vi "Drive Controller.vi"(8 "error in":errorcluster) -> ()   [LabVIEW 2016]
doc: "This VI executes continuously carrying out the current operation and responding to updates or new operation requests. It will often contain the timing or control code that is difficult to place directly in TeleOp. This VI generally opens all sensors and motors and isolates the rest of the robot code from knowing implementation details of how the operations are carried out."
uses:
  Drive Setpoints.ctl
  Drive Operations.ctl
  <vilib>/Rock Robotics/WPI/SafetyOutput/WPI_SafetyOutputConfigMenu.ctl
  <vilib>/Rock Robotics/WPI/Solenoid/WPI_SolenoidChannel.ctl
  <vilib>/Rock Robotics/SystemInterfaces/DIO/FPGA_DIOChannel.ctl
  <vilib>/Rock Robotics/WPI/ThirdParty/CanMotor/TalonSRX/WPI_CANTalonSRX_APIControlMode.ctl
  <vilib>/Rock Robotics/SystemInterfaces/AI/FPGA_AIChannel.ctl
  <vilib>/Rock Robotics/SystemInterfaces/spilib/spi_bus.ctl
  <vilib>/Rock Robotics/WPI/Solenoid/WPI_SolenoidValue.ctl
  <vilib>/Rock Robotics/WPI/Solenoid/WPI_SolenoidOpenDouble.vi
  <vilib>/Rock Robotics/WPI/Counter/WPI_CounterDigitalInputToDigitalSource.vi
  <vilib>/Rock Robotics/WPI/RobotDrive/WPI_RobotDriveOpen2MotorWithExistingMotors.vi
  <vilib>/Rock Robotics/WPI/Solenoid/WPI_SolenoidOpenSingle.vi
  <vilib>/Rock Robotics/WPI/ThirdParty/Sensors/Pigeon IMU/CTRE_PigeonIMU_Open_CAN.vi
  <vilib>/Rock Robotics/Network Tables/NT Read Number.vi
  <vilib>/Rock Robotics/WPI/Solenoid/WPI_SolenoidSetEnum.vi
  Drive Published Globals.vi
  <vilib>/Rock Robotics/Network Tables/NT Write Boolean.vi
  <vilib>/Rock Robotics/Network Tables/NT Write Number.vi
  Framework/Robot Global Data.vi
  <vilib>/addons/control/pid/pid.llb/PID (DBL).vi
  <vilib>/Rock Robotics/Network Tables/NT Write String.vi
  <vilib>/addons/control/pid/NI_PID_pid.lvlib
  <vilib>/Rock Robotics/WPI/ThirdParty/Sensors/navX/_Processing Loop/FRIC_navX_Internal_I2C_ProcessingLoop.vi
panel:
  out "Pigeon  Chart 2":dbl(graph)=-34.541015625
  out "Voltage now":dbl=1.910400195
  in  "Fcurving right":dbl=0.0045 format="%#_13g"
  in  "Fcurving left":dbl=0.0045 format="%#_13g"
  out "Vision P tuning threshold":dbl(graph)=6.5
  in  "AverageBits":u8=20
  out "Voltage Graph":dbl(graph)=1.910400195
  out "Voltage":dbl=1.2902830710000002
  in  "Threshold voltage":dbl=1.8
  out "Waveform Chart 2":cluster{"Heading":dbl, "\n\n\npigeon":dbl}(graph)={"Heading"=81.826171875, "\n\n\npigeon"=39.0673828125}
  out "Pigeon angle":dbl
  out "Waveform Chart":cluster{"Distance":dbl, "Distance":dbl}(graph)={"Distance"=9964.75, "Distance"=10153.75}
  in  "PDriveStright":dbl=0.02
  out "Pigeon  Chart":dbl(graph)=-40.1220703125
  in  "P curving factor":dbl=2.0
  in  "Theshold for curve":dbl=9.0
  in  "X resolution":dbl=160.0
  in  "y":dbl=0.15
  in  "PID gains":T1={"proportional gain (Kc)"=0.1, "integral time (Ti, min)"=0.0, "derivative time (Td, min)"=0.0} {"derivative time (Td, min)" format="%.3f"; "integral time (Ti, min)" format="%.3f"; "proportional gain (Kc)" format="%.3f"}
  in  "Score Cutoff":dbl=40.0
  in  "Y stopping threshold":dbl=70.0
  in  "ticks per rotation":dbl=512.0
  in  "Base Speed":dbl=-0.5499999999999999
  in  "P Gear Tuner":dbl=0.5
  in  "Max dist":dbl=1.0
  out "Setpoints":T2(graph)
  out "Current\nCmd":string="Started at  12:31:04.564\nDefault: Reserve,  L 0.0, R 0.0, D 0.000000"
  # "Gear Vision Stuff"
  # "Tip: It may be helpful to observe inputs and sensor values.\nYou may also want to display tuning or debugging controls."
  # "Used to be .25 on comp robot, .3 may work better though"
  # ".02*10 degrees =.2 motor power!!!"
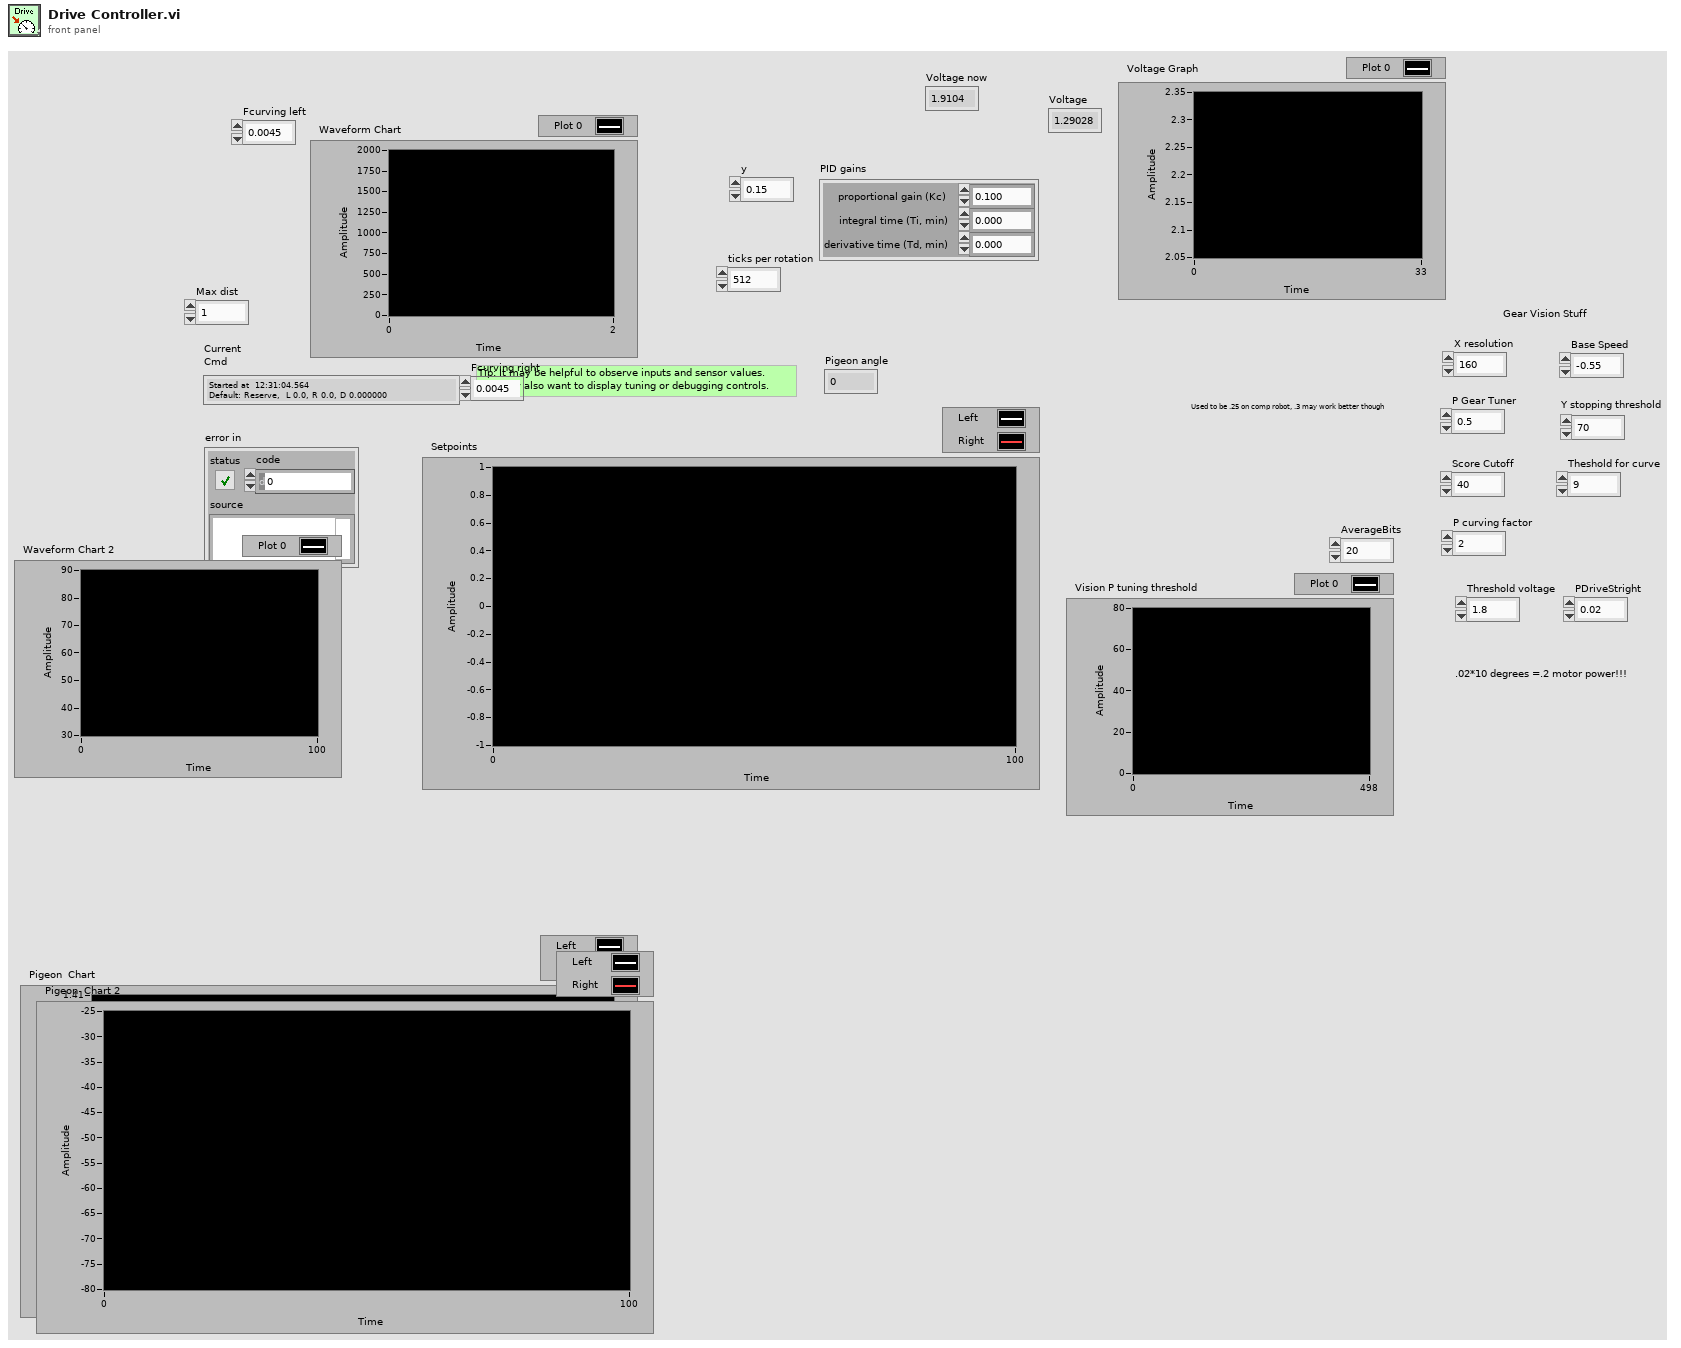
[diagram p1: front panel]
types:
  T1 = cluster{"proportional gain (Kc)":dbl, "integral time (Ti, min)":dbl, "derivative time (Td, min)":dbl}
  T2 = cluster{"Left Setpoint":dbl, "Right Setpoint":dbl}
  T3 = typedef "FPGA_AIChannel.ctl" = enum8{"AI 0", "AI 1", "AI 2", "AI 3", "AI MXP 0", "AI MXP 1", "AI MXP 2", "AI MXP 3", "Invalid"}
  T4 = typedef "WPI_SolenoidChannel.ctl" = enum8{"Solenoid 0", "Solenoid 1", "Solenoid 2", "Solenoid 3", "Solenoid 4", "Solenoid 5", "Solenoid 6", "Solenoid 7", "Invalid"}
  T5 = typedef "WPI_CANTalonSRX_APIControlMode.ctl" = enum8{"Percent VBus", "Speed", "Position", "Slave", "Unchanged / Invalid", "Voltage Compensation", "Current", "Motion Profile", "Motion Magic"}
  T6 = typedef "FPGA_DIOChannel.ctl" = enum8{"DIO 0", "DIO 1", "DIO 2", "DIO 3", "DIO 4", "DIO 5", "DIO 6", "DIO 7", "DIO 8", "DIO 9", "DIO MXP 0", "DIO MXP 1", "DIO MXP 2", "DIO MXP 3", "DIO MXP 4", "DIO MXP 5", "DIO MXP 6", "DIO MXP 7", "DIO MXP 8", "DIO MXP 9", "DIO MXP 10", "DIO MXP 11", "DIO MXP 12", "DIO MXP 13", "DIO MXP 14", "DIO MXP 15", "SPI Port CS1", "SPI Port CS2", "SPI Port CS3", "SPI Port MISO", "SPI Port MOSI", "Invalid"}
  T7 = typedef "spi_bus.ctl" = enum16{"SPI On-Board, CS0", "SPI On-Board, CS1", "SPI On-Board, CS2", "SPI On-Board, CS3", "SPI MXP", "Invalid"}
  T8 = typedef "WPI_SafetyOutputConfigMenu.ctl" = enum16{"Enable", "Disable"}
  T9 = typedef "Drive Setpoints.ctl" = cluster{"Operation":T10, "Left Setpoint":dbl, "Right Setpoint":dbl, "Duration":dbl, "Shift state":i8, "Angle":dbl, "Brake":bool}
  T10 = typedef "Drive Operations.ctl" = enum16{"Reserve", "Read Current", "Immediate", "Drive for Time", "Drive for Distance", "Turn to angle", "Vision Turn", "Vision close distance", "Reset Gyro", "Turn until target", "Brake", "One side PID drive straight", "turn to zero", "DriveStraight"}
  T11 = typedef "WPI_DigitalInputDevRef.ctl" = cluster{"DevStatus":errorcluster, "DIO Channel":T6}
  T12 = typedef "WPI_MotorControlDeviceRef.ctl" = cluster{"DeviceStatus":errorcluster, "Type":T13, "PWM":cluster{"PWM Channel":T14, "DeadBand":T15}, "CAN":cluster{"Device Number":u8, "SetOutput VI Ref":variant, "GetOutput VI Ref":variant, "Enable VI Ref":variant, "Disable VI Ref":variant, "Data":variant}, "Invert":bool}
  T13 = typedef "WPI_MotorControlType.ctl" = enum16{"PWM", "CAN"}
  T14 = typedef "FPGA_DIOPWMChannel.ctl" = enum8{"PWM 0", "PWM 1", "PWM 2", "PWM 3", "PWM 4", "PWM 5", "PWM 6", "PWM 7", "PWM 8", "PWM 9", "PWM MXP 0", "PWM MXP 1", "PWM MXP 2", "PWM MXP 3", "PWM MXP 4", "PWM MXP 5", "PWM MXP 6", "PWM MXP 7", "PWM MXP 8", "PWM MXP 9", "Invalid"}
  T15 = typedef "WPI_PWMDeadband.ctl" = cluster{"Name":string, "maxPositivePwm":i32, "minPositivePwm":i32, "centerPwm":i32, "maxNegativePwm":i32, "minNegativePwm":i32, "angularRange":u16}
  T16 = typedef "WPI_RobotDriveDevRef.ctl" = cluster{"DevStatus":errorcluster, "Motors[]":T12[], "Square Inputs":bool, "Max Output":dbl}
  T17 = typedef "FPGA_CounterEncoderSourceConvertionLVSourceType.ctl" = cluster{"DevStatus":errorcluster, "AnalogTriggerMode?":bool, "DigitalMode":cluster{"DIO Channel":T18}, "AnalogTriggerMode":cluster{"AnalogTriggerIndex":T19, "OutputType":T20}}
  T18 = typedef "FPGA_DIODigitalSourceChannel.ctl" = enum8{"DIO 0", "DIO 1", "DIO 2", "DIO 3", "DIO 4", "DIO 5", "DIO 6", "DIO 7", "DIO 8", "DIO 9", "DIO MXP 0", "DIO MXP 1", "DIO MXP 2", "DIO MXP 3", "DIO MXP 4", "DIO MXP 5", "DIO MXP 6", "DIO MXP 7", "DIO MXP 8", "DIO MXP 9", "DIO MXP 10", "DIO MXP 11", "DIO MXP 12", "DIO MXP 13", "DIO MXP 14", "DIO MXP 15", "Disabled"}
  T19 = typedef "FPGA_AnalogTriggerIndex.ctl" = enum8{"Trig 0", "Trig 1", "Trig 2", "Trig 3", "Trig 4", "Trig 5", "Trig 6", "Trig 7", "Invalid"}
  T20 = typedef "FPGA_AnalogTriggerOutType.ctl" = enum16{"InWindow", "TriggerState", "Rising", "Falling"}
  T21 = typedef "WPI_EncoderDevRef.ctl" = cluster{"DevStatus":errorcluster, "EncoderIndex":T22, "CounterIndex":T23, "DistancePerCount":dbl, "Decoding Type":T24}
  T22 = typedef "FPGA_EncoderIdx.ctl" = enum8{"Enc 0", "Enc 1", "Enc 2", "Enc 3", "Enc 4", "Enc 5", "Enc 6", "Enc 7", "Invalid"}
  T23 = typedef "FPGA_CounterCtrSystemIndex.ctl" = enum8{"Ctr 0", "Ctr 1", "Ctr 2", "Ctr 3", "Ctr 4", "Ctr 5", "Ctr 6", "Ctr 7", "Invalid"}
  T24 = typedef "WPI_EncoderType.ctl" = enum16{"1x", "2x", "4x"}
  T25 = typedef "WPI_SolenoidDevRef.ctl" = cluster{"DevStatus":errorcluster, "Pneumatics Control Module":u8, "Forward Solenoid Channel":T4, "Reverse Solenoid Channel":T4}
  T26 = typedef "Command Status Info.ctl" = cluster{"Name":string, "Status":T27, "notifier out":T28}
  T27 = typedef "Completion Status.ctl" = enum16{"Successful", "Aborted", "Incomplete"}
  T28 = typedef "Completion Notifier.ctl" = refnum<notifier>
  T29 = cluster{"SubSystem Data":T9, cluster{"Start Time (ms)":u32, "Iterations":i32}, cluster{"Command Info":T26, "Description":string, "SubSystem Data":T9, "notifier out":refnum<notifier>, "Subsystem Name":string}}
  T30 = typedef "CTRE_PigeonIMU_DeviceRef.ctl" = cluster{"DeviceStatus":errorcluster, "Device Number":u8, "Type":T31, "Device ID":u32}
  T31 = typedef "CTRE_PigeonIMU_ConnectionType.ctl" = u32
  T32 = typedef "WPI_AnalogChannelDevRef.ctl" = cluster{"DevStatus":errorcluster, "Analog Channel":T3}
  T33 = typedef "WPI_SolenoidValue.ctl" = enum16{"Off", "On", "Forward", "Reverse"}
  T34 = typedef "CTRE_PigeonIMU_GlobalStatus.ctl" = cluster{"PigeonState":T35, "FusedHeading":cluster{"Heading":dbl, "Valid?":bool, "Fusing?":bool}, "YPR":cluster{"Yaw":dbl, "Pitch":dbl, "Roll":dbl}, "Compass":cluster{"Heading":dbl, "Magnitude":dbl, "Absolute Heading":dbl}, "Accelerometer":cluster{"Biased":cluster{"X":i16, "Y":i16, "Z":i16, "Norm":i16}, "Angles":cluster{"XZ Tilt":dbl, "YZ Tilt":dbl, "XY Tilt":dbl}}, "Magnetometer":cluster{"Raw":cluster{"X":i16, "Y":i16, "Z":i16}, "Biased":cluster{"X":i16, "Y":i16, "Z":i16}}, "Gyro":cluster{"X":dbl, "Y":dbl, "Z":dbl, "Norm":dbl}, "6D Quaternian":cluster{"W":dbl, "X":dbl, "Y":dbl, "Z":dbl}, "Temp. (C)":dbl, "UpTime":u32, "StartupStatus":cluster{"ResetCount":i32, "ResetFlags":i32, "FirmwareVersion":i32, "HasReset?":bool}, "Calibration":cluster{"CurrentMode":T36, "LastCalError":i32, "CalBooting?":bool}, "CAN Error":errorcluster, "AccumGyro":cluster{"X":dbl, "Y":dbl, "Z":dbl}, "Usage Frame":u32}
  T35 = typedef "CTRE_PigeonIMU_PigeonState.ctl" = enum16{"NoComm", "Initializing", "Ready", "UserCalibration"}
  T36 = typedef "CTRE_PigeonIMU_CalibrationMode.ctl" = u16
  T37 = cluster{"Left":dbl, "Top":dbl, "Right":dbl, "Bottom":dbl}
  T38 = cluster{"SubSystem Data":T9, cluster{"Start Time (ms)":u32, "Iterations":i32}, "Default Command Arguments":cluster{"Command Info":T26, "Description":string, "SubSystem Data":T9, "notifier out":refnum<notifier>, "Subsystem Name":string}}
  T39 = typedef "WPI_DriverStationRobotMode2.ctl" = enum16{"Autonomous Disabled", "Autonomous Enabled", "Teleop Disabled", "Teleop Enabled", "Disconnected", "Finish", "Test Disabled", "Test Enabled", "Emergency Stopped"}
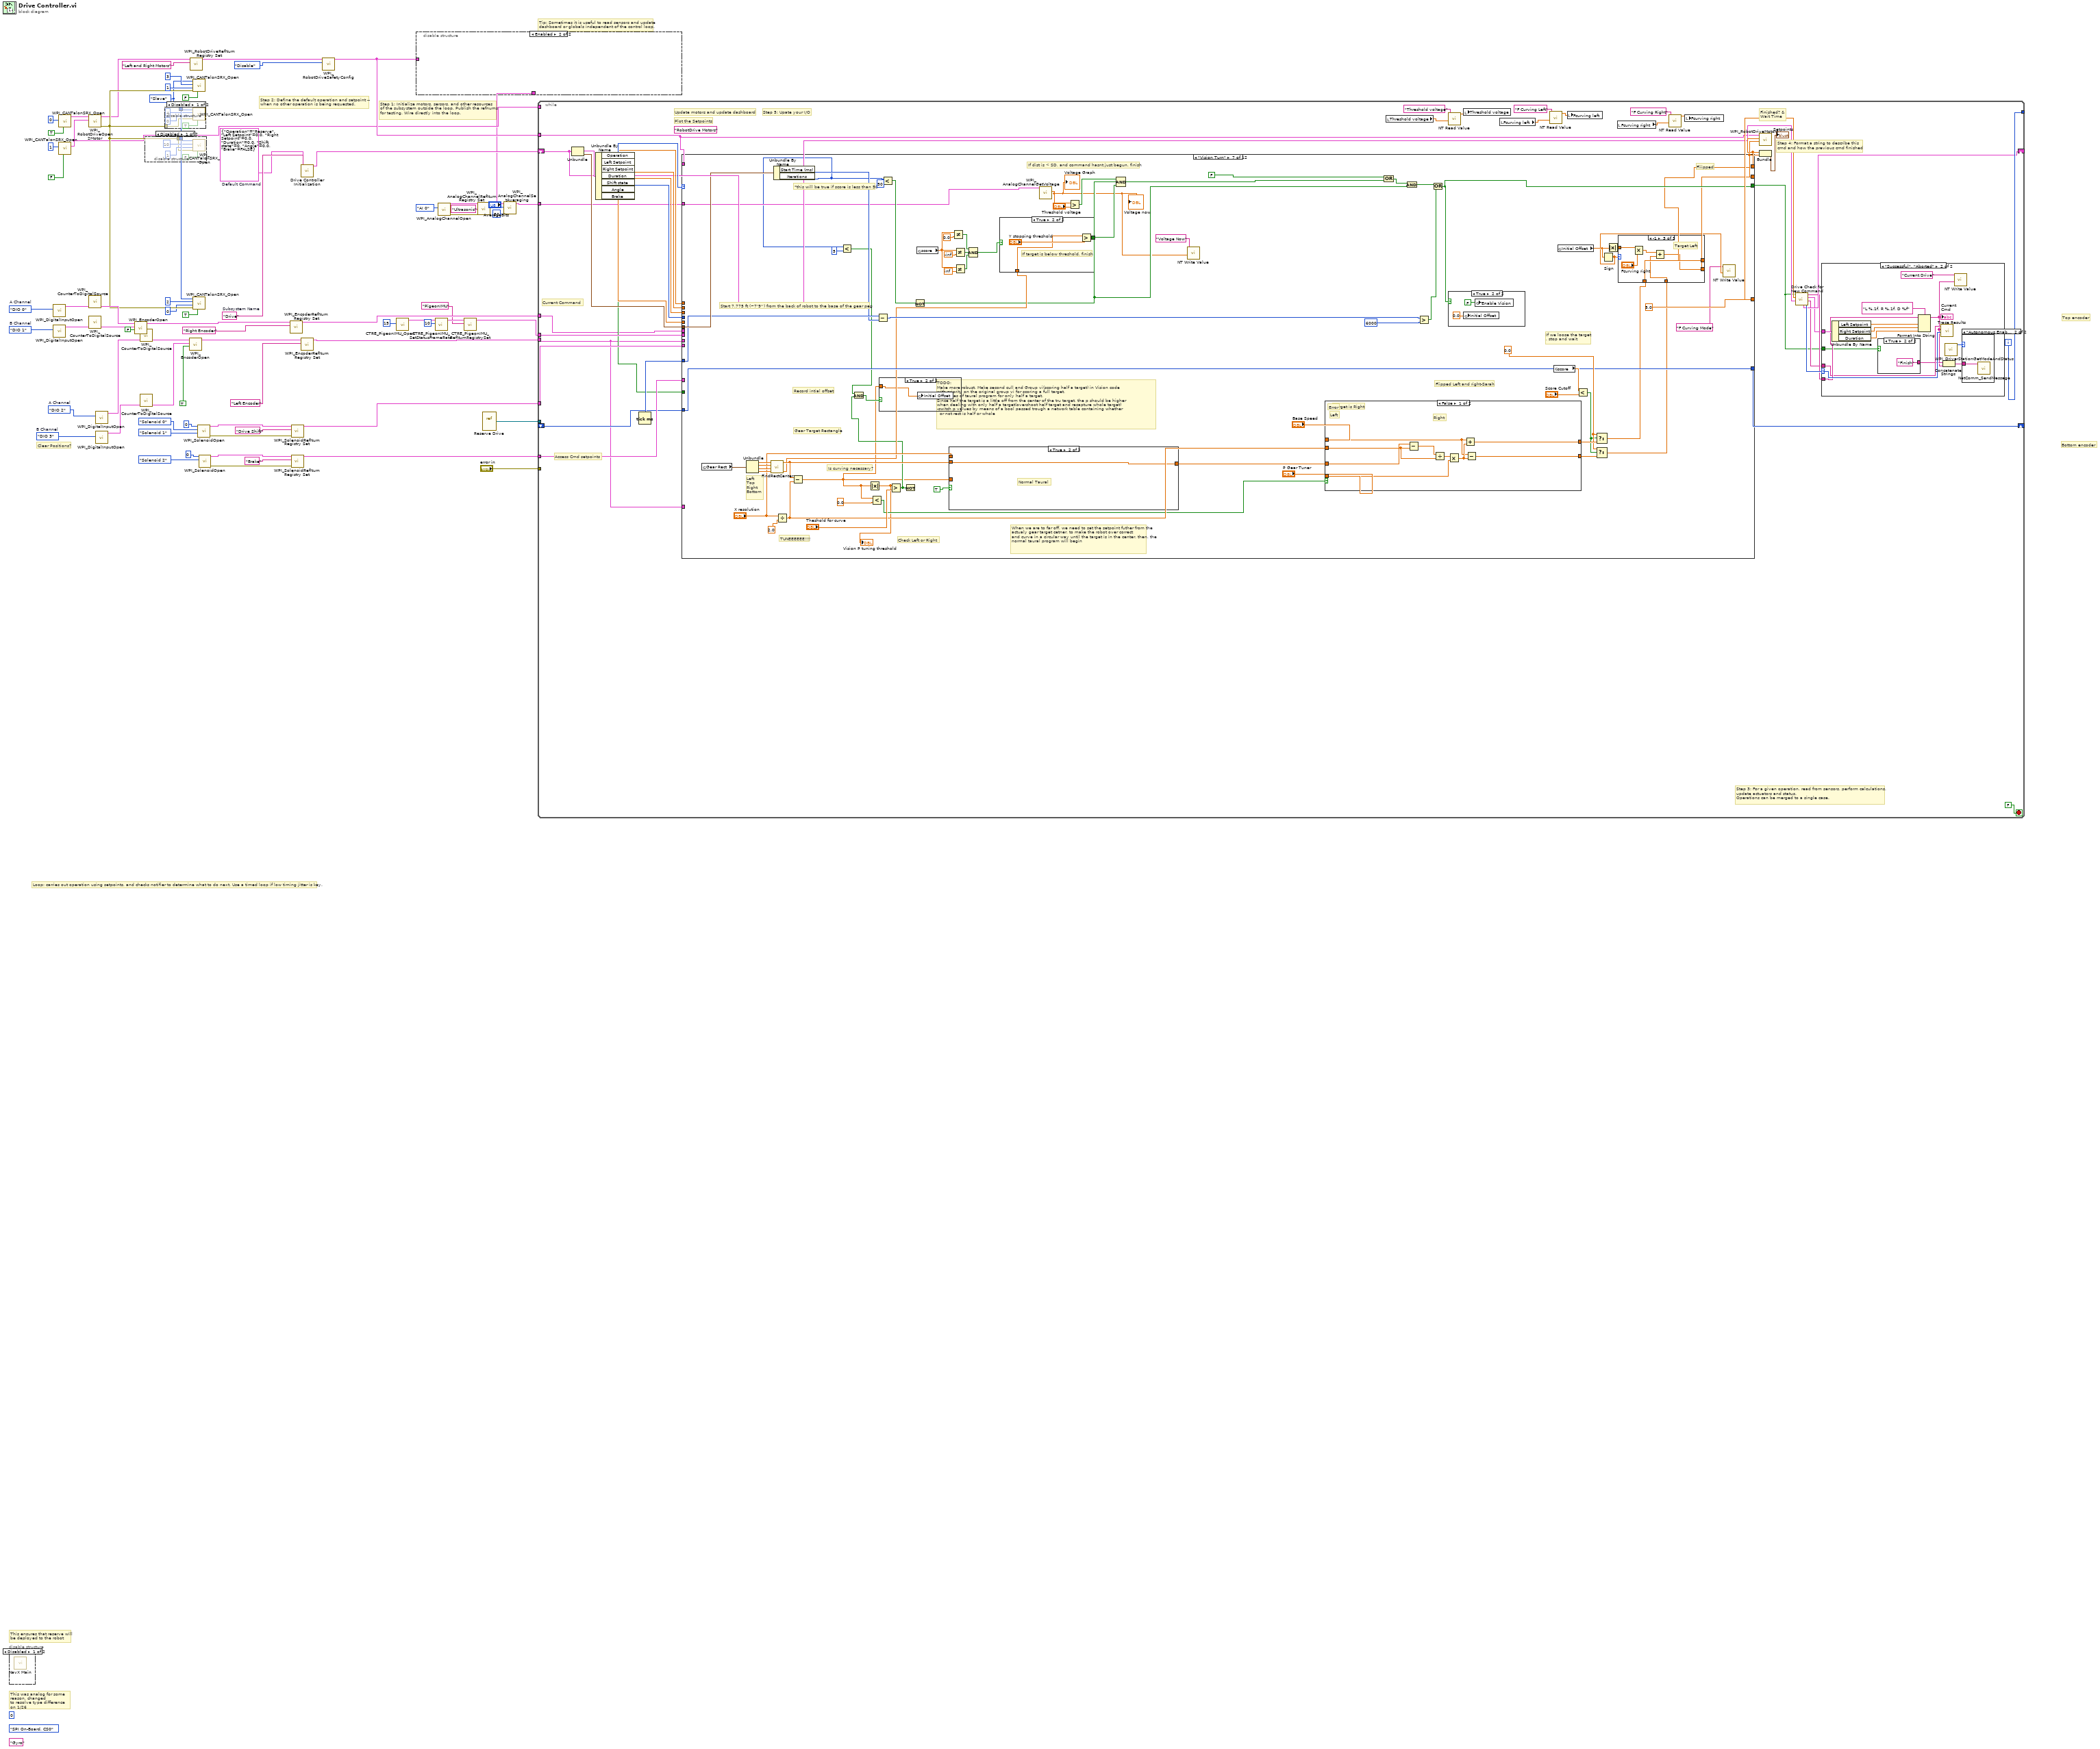
[diagram p0: block diagram]
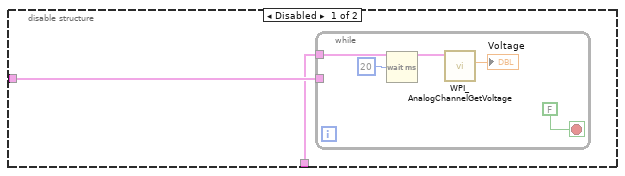
[diagram p5: hidden frame]
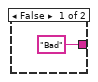
[diagram p7: hidden frame]
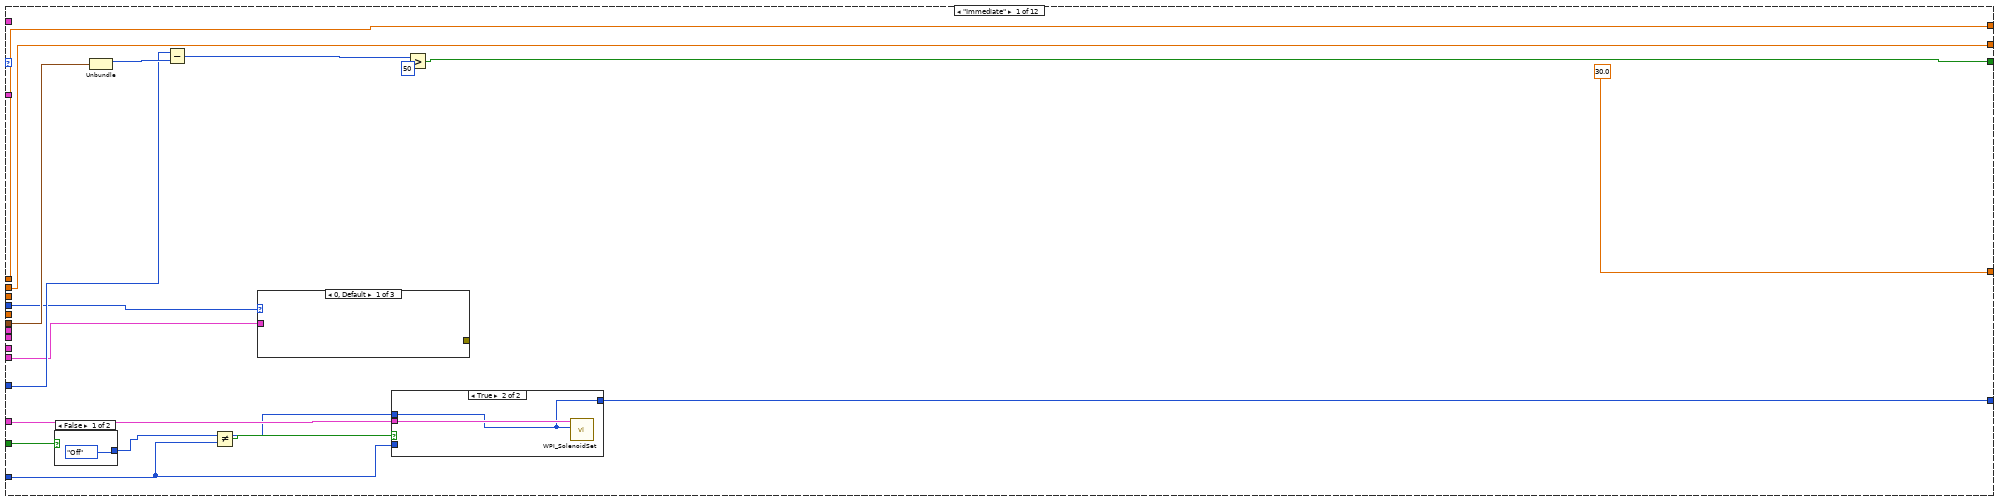
[diagram p9: hidden frame]
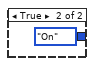
[diagram p10: hidden frame]
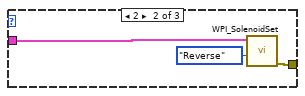
[diagram p12: hidden frame]
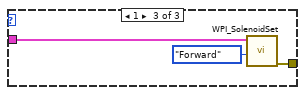
[diagram p13: hidden frame]
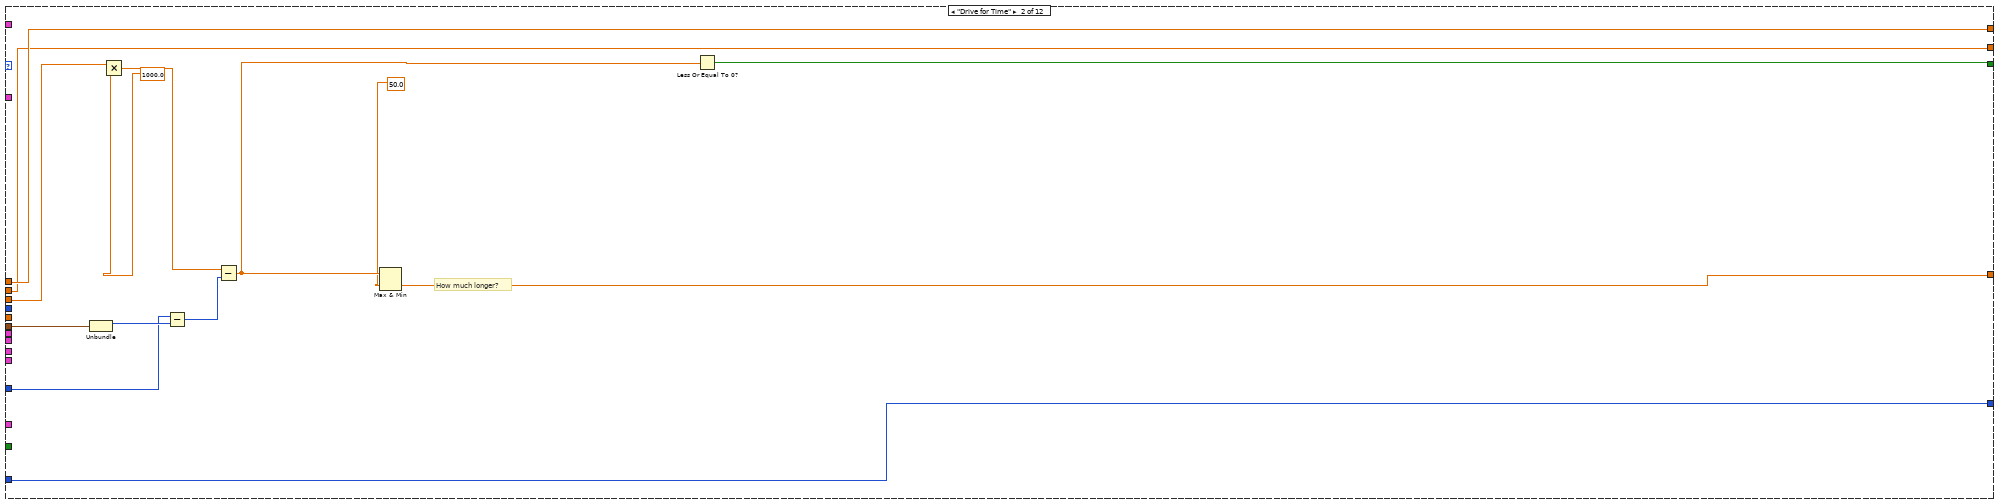
[diagram p14: hidden frame]
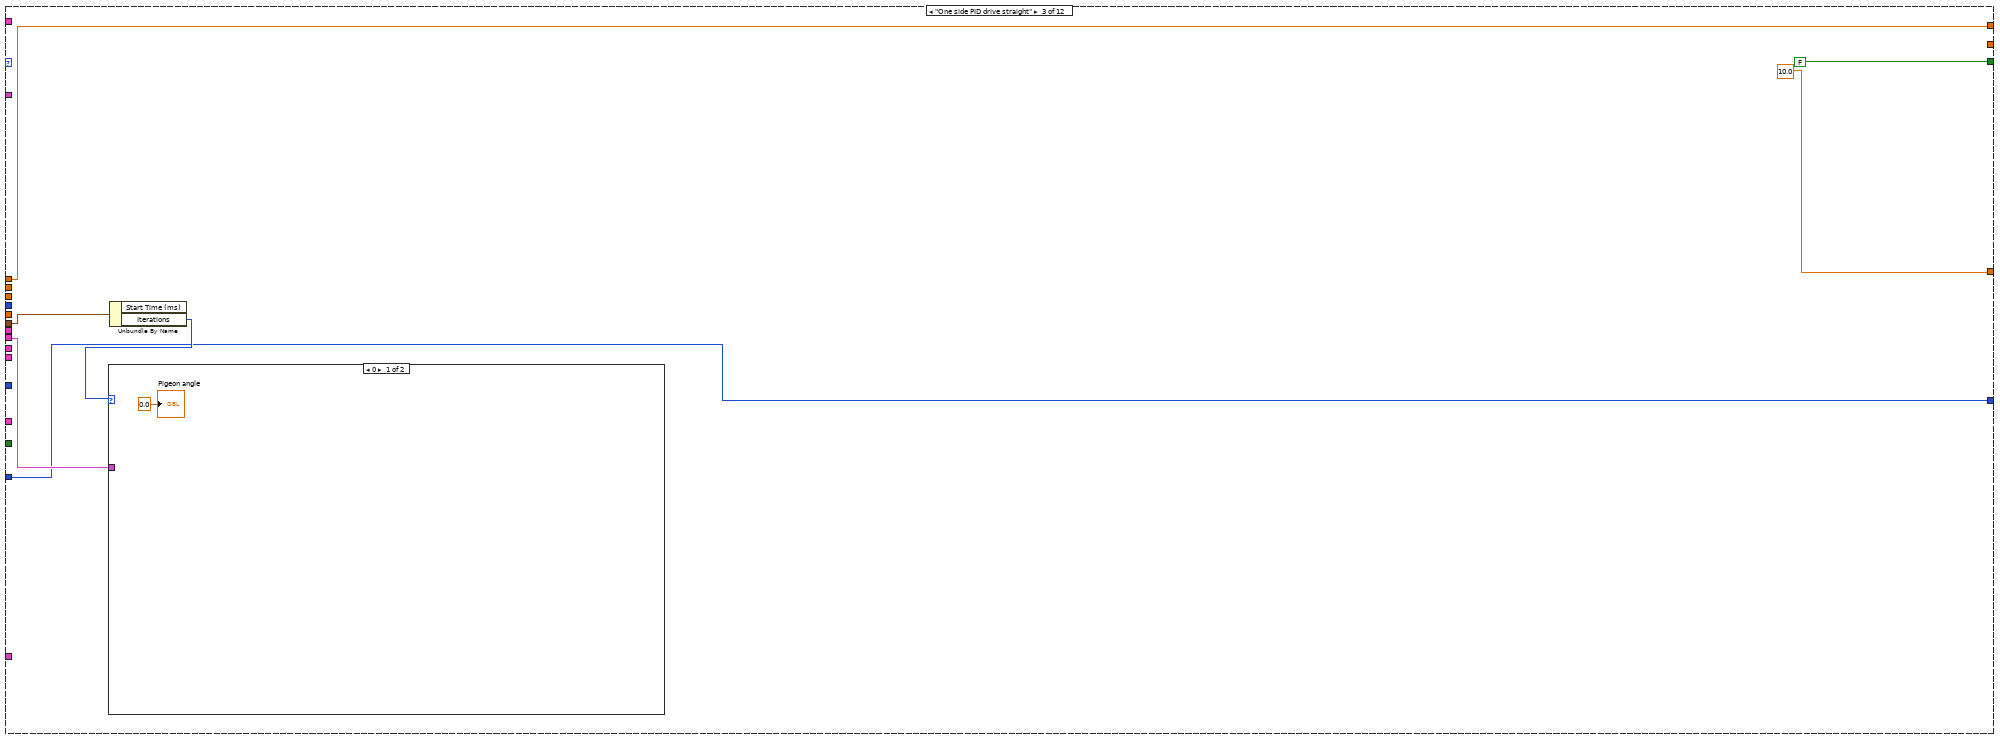
[diagram p15: hidden frame]
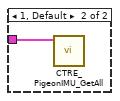
[diagram p16: hidden frame]
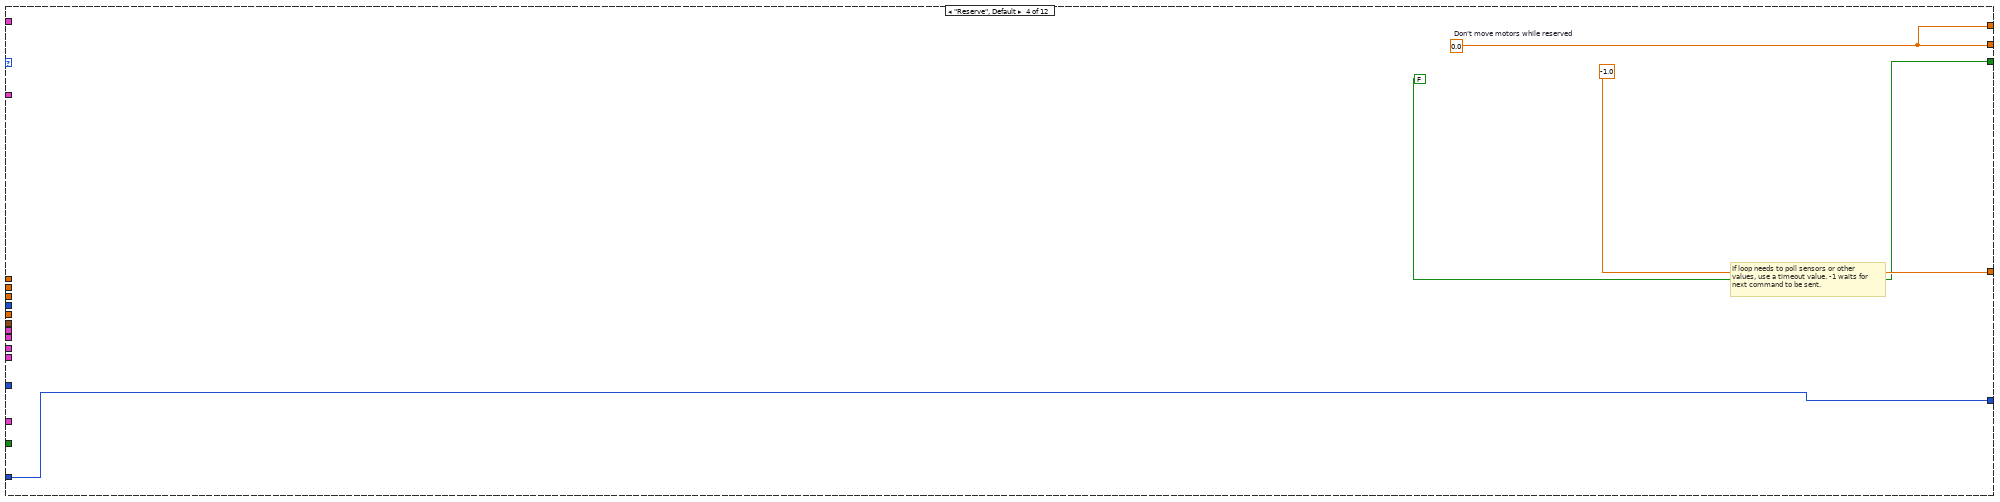
[diagram p17: hidden frame]
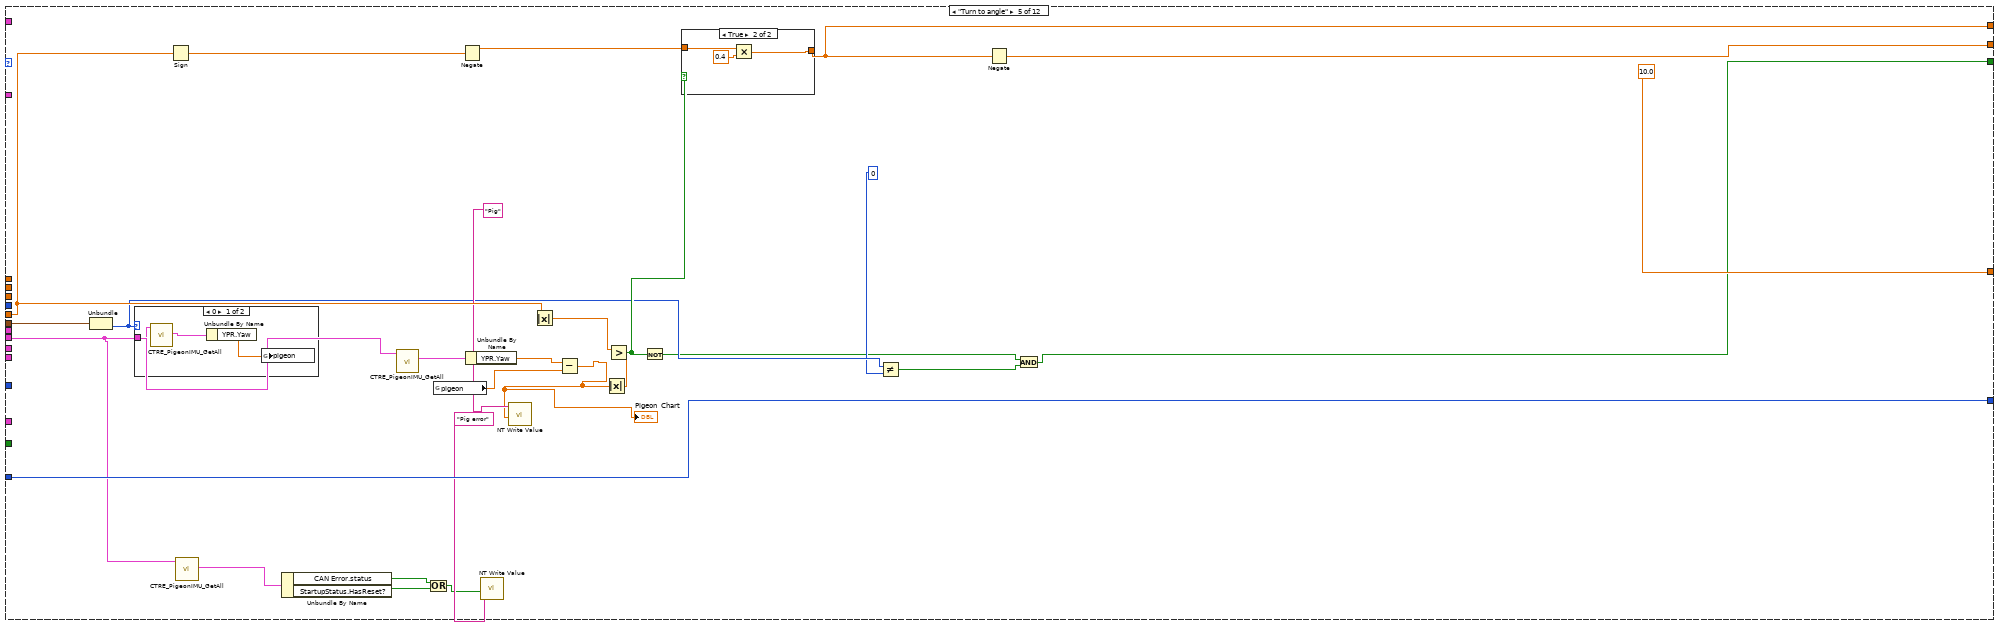
[diagram p18: hidden frame]
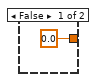
[diagram p20: hidden frame]
diagram:
  w25 = WPI_CANTalonSRX_APIControlMode."Slave" ("Control Mode")
  w51 = FPGA_DIOChannel."DIO 3"  # B Channel
  w50 = FPGA_DIOChannel."DIO 2"  # A Channel
  w56 = FPGA_DIOChannel."DIO 1"  # B Channel
  w55 = FPGA_DIOChannel."DIO 0"  # A Channel
  (unwired) spi_bus."SPI On-Board, CS0" ("SPI Bus")
  (unwired) "Gyro" ("refnum name")
  (unwired) u8 0 ("Rear Left Motor")
  w70 = T9 {"Operation"=enum."Reserve", "Left Setpoint"=0.0, "Right Setpoint"=0.0, "Duration"=0.0, "Shift state"=0, "Angle"=0.0, "Brake"=FALSE}  # Default Command
  w71 = "Drive"  # Subsystem Name
  # "Bottom encoder"
  # "Top encoder"
  # "Clear Positions?"
  # "This was analog for some reason, changed \nto resolve type difference \non 1/26"
  # "This ensures that reserve will\nbe deployed to the robot"
  # "Tip: Sometimes it is useful to read sensors and update\ndashboard or globals independent of the control loop."
  # "Step 2: Define the default operation and setpoint --\nwhen no other operation is being requested."
  # "Step 1: Initialize motors, sersors, and other resources\nof the subsystem outside the loop. Publish the refnums\nfor testing. Wire directly into the loop."
  # "Loop: carries out operation using setpoints, and checks notifier to determine what to do next. Use a timed loop if low timing jitter is key."
  n1 = disable-structure shown="Disabled" {
    frame Disabled {
      n2 = call-poly <vilib>:"NavX Main.vi"() -> ()  [unwired: 12 in]
    }
    frame Enabled {
    }
  }
  n3 = call <vilib>:"WPI_DigitalInputOpen.vi"("DIO Channel"=w55) -> ("DigitalInputDevRef"=w52:T11)  [unwired: 1 in, 9 out]
  n4 = call <vilib>:"WPI_DigitalInputOpen.vi"("DIO Channel"=w56) -> ("DigitalInputDevRef"=w53:T11)  [unwired: 1 in, 9 out]
  n5 = call <vilib>:"WPI_CANTalonSRX_Open.vi"("Invert"=TRUE, "Device Number"=u8 0) -> ("CAN Talon SRX Ref"=w30:T12)  [unwired: 8 in, 1 out]
  n6 = call <vilib>:"WPI_CANTalonSRX_Open.vi"("Invert"=FALSE, "Device Number"=u8 1) -> ("CAN Talon SRX Ref"=w9:T12)  [unwired: 8 in, 1 out]
  n7 = call-poly <vilib>:"WPI_RobotDriveOpen2Motor.vi"("Right Motor Dev Ref"=w9, "Left Motor Dev Ref"=w30) -> ("error out"=w29:errorcluster, "RobotDriveDevRef"=w26:T16)  [unwired: 8 in]
  n8 = call-poly <vilib>:"WPI_CounterToDigitalSource.vi"("DigitalInputDevRef"=w52) -> ("Digital Source"=w45:T17)  [unwired: 6 out]
  n9 = call-poly <vilib>:"WPI_CounterToDigitalSource.vi"("DigitalInputDevRef"=w53) -> ("Digital Source"=w54:T17)  [unwired: 6 out]
  n10 = call <vilib>:"WPI_DigitalInputOpen.vi"("DIO Channel"=w50) -> ("DigitalInputDevRef"=w47:T11)  [unwired: 1 in, 9 out]
  n11 = call <vilib>:"WPI_DigitalInputOpen.vi"("DIO Channel"=w51) -> ("DigitalInputDevRef"=w48:T11)  [unwired: 1 in, 9 out]
  n12 = call <vilib>:"WPI_EncoderOpen.vi"("Invert Direction (False)"=FALSE, "BSource"=w54, "ASource"=w45) -> ("EncoderDevRef"=w44:T21)  [unwired: 5 in, 3 out]
  n13 = call-poly <vilib>:"WPI_CounterToDigitalSource.vi"("DigitalInputDevRef"=w47) -> ("Digital Source"=w46:T17)  [unwired: 6 out]
  n14 = call-poly <vilib>:"WPI_CounterToDigitalSource.vi"("DigitalInputDevRef"=w48) -> ("Digital Source"=w49:T17)  [unwired: 6 out]
  n15 = disable-structure shown="Disabled" {
    disable-tunnel: w29 -> [w73 _]
    disable-tunnel: w25 -> [w72 _]
    frame Disabled {
      n16 = call <vilib>:"WPI_CANTalonSRX_Open.vi"("Invert"=FALSE, "error in"=w73, "Master Device Number"=u8 1, "Device Number"=u8 10, "Control Mode"=w72) -> ()  [unwired: 5 in, 2 out]
    }
    frame Enabled {
    }
  }
  n17 = disable-structure shown="Disabled" {
    disable-tunnel: w29 -> [w78 _]
    disable-tunnel: w25 -> [w77 _]
    frame Disabled {
      n18 = call <vilib>:"WPI_CANTalonSRX_Open.vi"("Invert"=TRUE, "error in"=w78, "Master Device Number"=u8 0, "Device Number"=u8 4, "Control Mode"=w77) -> ()  [unwired: 5 in, 2 out]
    }
    frame Enabled {
    }
  }
  n19 = call <vilib>:"WPI_EncoderOpen.vi"("Invert Direction (False)"=TRUE, "BSource"=w49, "ASource"=w46) -> ("EncoderDevRef"=w41:T21)  [unwired: 5 in, 3 out]
  n20 = call <vilib>:"WPI_RobotDriveRefNum Registry Set.vi"("refnum name"="Left and Right Motors", "RobotDriveDevRef"=w26) -> ("RobotDriveDevRef"=w68:T16)  [unwired: 2 in, 7 out]
  n21 = call <vilib>:"WPI_CANTalonSRX_Open.vi"("Invert"=FALSE, "error in"=w29, "Master Device Number"=u8 1, "Device Number"=u8 3, "Control Mode"=w25) -> ()  [unwired: 5 in, 2 out]
  n22 = call <vilib>:"WPI_CANTalonSRX_Open.vi"("Invert"=TRUE, "error in"=w29, "Master Device Number"=u8 0, "Device Number"=u8 2, "Control Mode"=w25) -> ()  [unwired: 5 in, 2 out]
  n23 = call-poly <vilib>:"WPI_SolenoidOpen.vi"("Reverse Solenoid Channel"=WPI_SolenoidChannel."Solenoid 1", "Forward Solenoid Channel"=WPI_SolenoidChannel."Solenoid 0", "Pneumatics Control Module (0)"=u8 0) -> ("error out"=w57:errorcluster, "SolenoidDevRef"=w59:T25)  [unwired: 7 in]
  n24 = call-poly <vilib>:"WPI_SolenoidOpen.vi"("Solenoid Channel"=WPI_SolenoidChannel."Solenoid 2" ("Forward Solenoid Channel"), "Pneumatics Control Module (0)"=u8 0) -> ("error out"=w19:errorcluster, "SolenoidDevRef"=w22:T25)  [unwired: 8 in]
  n25 = call <vilib>:"WPI_EncoderRefNum Registry Set.vi"("refnum name"="Right Encoder", "EncoderDevRef"=w44) -> ("EncoderDevRef"=w43:T21)  [unwired: 8 in, 1 out]
  n26 = call <vilib>:"WPI_SolenoidRefNum Registry Set.vi"("error in (no error)"=w57, "refnum name"="Drive Shift", "SolenoidDevRef"=w59) -> ("SolenoidDevRef"=w14:T25)  [unwired: 7 in, 1 out]
  n27 = call <vilib>:"WPI_SolenoidRefNum Registry Set.vi"("error in (no error)"=w19, "refnum name"="Brake", "SolenoidDevRef"=w22) -> ("SolenoidDevRef"=w21:T25)  [unwired: 7 in, 1 out]
  n28 = call "Drive Controller Initialization.vi"("Subsystem Name"=w71, "Default Command"=w70) -> ("output cluster"=w64:T29)  [unwired: 9 in]
  n29 = call <vilib>:"WPI_EncoderRefNum Registry Set.vi"("refnum name"="Left Encoder", "EncoderDevRef"=w41) -> ("EncoderDevRef"=w40:T21)  [unwired: 8 in, 1 out]
  n30 = call <vilib>:"WPI_RobotDriveSafetyConfig.vi"("mode"=WPI_SafetyOutputConfigMenu."Disable", "RobotDriveDevRef"=w68) -> ("RobotDriveDevRef"=w66:T16)  [unwired: 8 in, 1 out]
  n31 = call-poly <vilib>:"CTRE_PigeonIMU_Open.vi"("Device Number"=u8 15) -> ("PigeonIMUDevRef"=w16:T30)  [unwired: 9 in, 1 out]
  n32 = call <vilib>:"CTRE_PigeonIMU_SetStatusFrameRate.vi"("Period (ms)"=i16 10, "PigeonIMUDevRef"=w16) -> ("PigeonIMUDevRef"=w15:T30)  [unwired: 8 in, 1 out]
  n33 = call <vilib>:"WPI_AnalogChannelOpen.vi"("Analog Channel"=FPGA_AIChannel."AI 0") -> ("error out"=w8:errorcluster, "AIDeviceRef"=w7:T32)  [unwired: 9 in]
  n34 = call <vilib>:"CTRE_PigeonIMU_RefNumRegistrySet.vi"("refnum name"="PigeonIMU", "PigeonIMUDevRef"=w15) -> ("PigeonIMUDevRef"=w13:T30)  [unwired: 8 in, 1 out]
  n35 = call <vilib>:"WPI_AnalogChannelRefNum Registry Set.vi"("error in (no error)"=w8, "refnum name"="Ultrasonic", "AIDeviceRef"=w7) -> ("AIDeviceRef"=w4:T32)  [unwired: 7 in, 1 out]
  n36 = disable-structure shown="Enabled" {
    disable-tunnel: w66 -> [w83 _]
    disable-tunnel: w4 -> [w82 _]
    frame Disabled {
      n37 = while {
        tunnel: w83 -> [_]
        tunnel: w82 -> [w84]
        stop <- FALSE stop-if-true
        n38 = Wait (ms)(milliseconds to wait=u32 20) -> ()  [unwired: 1 out]
        n39 = call <vilib>:"WPI_AnalogChannelGetVoltage.vi"("AIDeviceRef"=w84) -> ("Voltage"=→"Voltage":dbl)  [unwired: 8 in, 2 out]
      }
    }
    frame Enabled {
    }
  }
  n40 = vi-ref "Reserve Drive.vi"() -> (w63:refnum<vi>)
  n41 = call <vilib>:"WPI_AnalogChannelSetAveraging.vi"("OversampleBits"=u8 50, "AverageBits"="AverageBits", "AIDeviceRef"=w4) -> ("AIDeviceRef"=w3:T32)  [unwired: 7 in, 1 out]
  n42 = while {
    shift-right: [w116] -> _
    shift-left: w64 -> [w110]
    tunnel: [w127] -> _
    tunnel: w66 -> [w106]
    tunnel: "error in" -> [_]
    tunnel: w63 -> [_]
    tunnel: w14 -> [w108]
    tunnel: w43 -> [w89]
    tunnel: w40 -> [w88]
    tunnel: w21 -> [w105]
    tunnel: w13 -> [w104]
    shift-right: [w103] -> _
    shift-left: _ -> [w100]
    tunnel: w9 -> [_]
    tunnel: w3 -> [w99]
    i -> [w127]
    stop <- FALSE stop-if-true
    (unwired) "RobotDrive Motors" ("Name")
    # "Step 5: Upate your I/O"
    # "Step 4: Format a string to describe this\ncmd and how the previous cmd finished"
    # "Current Command"
    # "Update motors and update dashboard"
    # "Plot the Setpoints"
    # "Access Cmd setpoints"
    # "Finished? &\nWait Time"
    # "Step 3: For a given operation, read from sensors, perform calculations,\nupdate actuators and status.\nOperations can be merged to a single case."
    n43 = Unbundle(w110) -> ("SubSystem Data"=w123:T9, w111:cluster{"Start Time (ms)":u32, "Iterations":i32})  [unwired: 1 out]
    n44 = Unbundle By Name(w123) -> ("Operation"=w122:T10, "Left Setpoint"=w121:dbl, "Right Setpoint"=w120:dbl, "Duration"=w119:dbl, "Shift state"=w109:i8, "Angle"=w107:dbl, "Brake"=w102:bool)
    n45 = Tick Count (ms)() -> (millisecond timer value=w118:u32)
    n46 = case shown="\"Vision Turn\"" w122 {
      tunnel: [30.0 w175 10.0 -1.0 10.0 10.0 5.0 10.0 100.0 10.0 10.0 10.0] -> w115
      tunnel: [w158 w182 FALSE ("Distance Has Been Reached") FALSE ("ignore previous (F)") w201 w248 w301 w389 TRUE ("ignore previous (F)") w421 w461 w502] -> w101
      tunnel: w111 -> [w157 w184 w193 _ w224 w261 w320 _ _ w436 w483 _]
      tunnel: [w152 w181 w194 w198 w227 w264 w276 w394 _ w432 w462 w500] -> w125
      tunnel: [w151 w180 _ w198 w226 w263 w274 w393 _ w430 w462 w500] -> w124
      tunnel: w121 -> [w152 w181 w194 _ _ _ _ _ _ w412 w470 _]
      tunnel: w120 -> [w151 w180 _ _ _ _ _ _ _ w411 w481 _]
      tunnel: w119 -> [_ w179 _ _ _ _ _ _ _ w422 w487 _]
      tunnel: w118 -> [w159 w178 _ _ _ _ w315 _ _ _ _ _]
      tunnel: w109 -> [w156 _ _ _ _ _ _ _ _ _ _ _]
      tunnel: w108 -> [w155 _ _ _ _ _ _ _ _ _ _ _]
      tunnel: w107 -> [_ _ _ _ w220 _ _ _ _ _ _ _]
      tunnel: w106 -> [_ _ _ _ _ _ _ _ _ _ _ _]
      tunnel: w88 -> [_ _ _ _ _ _ _ _ _ w426 w478 _]
      tunnel: w105 -> [w148 _ _ _ _ _ _ _ w406 _ _ _]
      tunnel: w89 -> [_ _ _ _ _ _ _ _ _ w427 w479 _]
      tunnel: w104 -> [_ _ w191 _ w207 w246 _ _ _ w417 _ _]
      tunnel: [w153 w174 w189 w197 w218 w258 w316 w391 w405 w434 w480 w499] -> w103
      tunnel: w100 -> [w150 w174 w189 w197 w218 w258 w316 w391 _ w434 w480 w499]
      tunnel: w102 -> [w149 _ _ _ _ _ _ _ _ _ _ _]
      tunnel: w99 -> [_ _ _ _ _ _ w300 _ _ _ _ _]
      tunnel: w88 -> [_ _ _ _ _ _ _ _ _ _ _ _]
      frame "Immediate" {
        n47 = case shown="False" w149 {
          tunnel: [WPI_SolenoidValue."Off" ("Value") WPI_SolenoidValue."On" ("Value")] -> w147
          frame False {
          }
          frame True {
          }
        }
        n48 = Unbundle(w157) -> ("Start Time (ms)"=w160:u32)  [unwired: 1 out]
        n49 = Subtract(x=w159, y=w160) -> (x-y=w161:u32)
        n50 = Not Equal?(x=w147, y=w150) -> (x != y?=w154:bool)
        n51 = case shown="0, Default" w156 {
          tunnel: w155 -> [_ w169 w173]
          tunnel: [_ w168 w171] -> _
          frame 0, Default {
          }
          frame 2 {
            n52 = call-poly <vilib>:"WPI_SolenoidSet.vi"("Value"=WPI_SolenoidValue."Reverse", "SolenoidDevRef"=w169) -> ("error out"=w168:errorcluster)  [unwired: 8 in, 1 out]
          }
          frame 1 {
            n53 = call-poly <vilib>:"WPI_SolenoidSet.vi"("Value"=WPI_SolenoidValue."Forward", "SolenoidDevRef"=w173) -> ("error out"=w171:errorcluster)  [unwired: 8 in, 1 out]
          }
        }
        n54 = case shown="True" w154 {
          tunnel: [w165 w166] -> w153
          tunnel: w150 -> [w165 _]
          tunnel: w148 -> [_ w167]
          tunnel: w147 -> [_ w166]
          frame False {
          }
          frame True {
            n55 = call-poly <vilib>:"WPI_SolenoidSet.vi"("Value"=w166, "SolenoidDevRef"=w167) -> ()  [unwired: 8 in, 2 out]
          }
        }
        n56 = Greater?(x=w161, y=u8 50 ("Left Motor")) -> (0:w158:bool)
      }
      frame "Drive for Time" {
        # "How much longer?"
        n57 = Unbundle(w184) -> ("Start Time (ms)"=w183:u32)  [unwired: 1 out]
        n58 = Multiply(x=w179, y=1000.0) -> (x*y=w186:dbl)
        n59 = Subtract(x=w178, y=w183) -> (x-y=w187:u32)
        n60 = Subtract(x=w186, y=w187) -> (x-y=w177:dbl)
        n61 = Max & Min(x=w177, y=50.0) -> (min(x,y)=w175:dbl)  [unwired: 1 out]
        n62 = Less Or Equal To 0?(x=w177) -> (x <= 0?=w182:bool)
      }
      frame "One side PID drive straight" {
        n63 = Unbundle By Name(w193) -> ("Iterations"=w192:i32)  [unwired: 1 out]
        n64 = case shown="0" w192 {
          tunnel: w191 -> [_ w196]
          frame 0 {
            "Pigeon angle" <- 0.0 ("Pigeon angle")
          }
          frame 1, Default {
            n65 = call <vilib>:"CTRE_PigeonIMU_GetAll.vi"("PigeonIMUDevRef"=w196) -> ()  [unwired: 8 in, 3 out]
          }
        }
      }
      frame "Reserve", Default {
        w198 = 0.0  # Don't move motors while reserved
        # "If loop needs to poll sensors or other\nvalues, use a timeout value. -1 waits for\nnext command to be sent."
      }
      frame "Turn to angle" {
        n66 = Unbundle(w224) -> ("Iterations"=w205:i32)  [unwired: 1 out]
        n67 = case shown="0" w205 {
          tunnel: w207 -> [w228 _]
          frame 0 {
            n68 = call <vilib>:"CTRE_PigeonIMU_GetAll.vi"("PigeonIMUDevRef"=w228) -> ("Get All"=w230:T34)  [unwired: 8 in, 2 out]
            n69 = Unbundle By Name(w230) -> ("YPR.Yaw"=w229:dbl)
            n70 = global write "Drive Published Globals.vi" "pigeon"(w229) -> ()
          }
          frame 1, Default {
          }
        }
        n71 = Sign(1:w220) -> (0:w221:dbl)
        n72 = call <vilib>:"CTRE_PigeonIMU_GetAll.vi"("PigeonIMUDevRef"=w207) -> ("Get All"=w212:T34)  [unwired: 8 in, 2 out]
        n73 = Unbundle By Name(w212) -> ("CAN Error.status"=w210:bool, "StartupStatus.HasReset?"=w211:bool)
        n74 = call <vilib>:"CTRE_PigeonIMU_GetAll.vi"("PigeonIMUDevRef"=w207) -> ("Get All"=w223:T34)  [unwired: 8 in, 2 out]
        n75 = Or(x=w210, y=w211) -> (x .or. y?=w208:bool)
        n76 = global read "Drive Published Globals.vi" "pigeon"() -> (w214:dbl)
        n77 = Negate(x=w221) -> (-x=w219:dbl)
        n78 = Unbundle By Name(w223) -> ("YPR.Yaw"=w213:dbl)
        n79 = call-poly <vilib>:"NT Write Value.vi"("Boolean"=w208, "Name"="Pig error") -> ()  [unwired: 9 in, 1 out]
        n80 = Absolute Value(x=w220) -> (abs(x)=w216:dbl)
        n81 = Subtract(x=w213, y=w214) -> (x-y=w206:dbl)
        "Pigeon  Chart" <- w206
        n82 = call-poly <vilib>:"NT Write Value.vi"("Numeric"=w206, "Name"="Pig") -> ()  [unwired: 9 in, 1 out]
        n83 = Absolute Value(x=w206) -> (abs(x)=w215:dbl)
        n84 = Greater?(x=w216, y=w215) -> (0:w222:bool)
        n85 = Not(x=w222) -> (.not. x?=w202:bool)
        n86 = case shown="True" w222 {
          tunnel: [0.0 w232] -> w227
          tunnel: w219 -> [_ w234]
          frame False {
          }
          frame True {
            n87 = Multiply(x=w234, y=0.4) -> (x*y=w232:dbl)
          }
        }
        n88 = Not Equal?(x=w205, y=0) -> (x != y?=w203:bool)
        n89 = Negate(x=w227) -> (-x=w226:dbl)
        n90 = And(x=w202, y=w203) -> (x .and. y?=w201:bool)
      }
      frame "turn to zero" {
        n91 = Unbundle(w261) -> ("Iterations"=w247:i32)  [unwired: 1 out]
        n92 = global read "Drive Published Globals.vi" "Start angle"() -> (w242:dbl)
        n93 = call <vilib>:"CTRE_PigeonIMU_GetAll.vi"("PigeonIMUDevRef"=w246) -> ("Get All"=w256:T34)  [unwired: 8 in, 2 out]
        n94 = Unbundle By Name(w256) -> ("CAN Error.status"=w254:bool, "StartupStatus.HasReset?"=w255:bool)
        n95 = call <vilib>:"CTRE_PigeonIMU_GetAll.vi"("PigeonIMUDevRef"=w246) -> ("Get All"=w260:T34)  [unwired: 8 in, 2 out]
        n96 = Or(x=w254, y=w255) -> (x .or. y?=w252:bool)
        n97 = Unbundle By Name(w260) -> ("YPR.Yaw"=w243:dbl)
        "Pigeon  Chart 2" <- w243
        n98 = Subtract(x=w242, y=w243) -> (x-y=w241:dbl)
        n99 = Sign(1:w241) -> (0:w245:dbl)
        n100 = Negate(x=w245) -> (-x=w244:dbl)
        n101 = call-poly <vilib>:"NT Write Value.vi"("Boolean"=w252, "Name"="Pig error") -> ()  [unwired: 9 in, 1 out]
        n102 = call-poly <vilib>:"NT Write Value.vi"("Numeric"=w243, "Name"="Pig") -> ()  [unwired: 9 in, 1 out]
        n103 = global read "Drive Published Globals.vi" "Start angle"() -> (w239:dbl)
        n104 = Absolute Value(x=w243) -> (abs(x)=w240:dbl)
        n105 = Absolute Value(x=w239) -> (abs(x)=w238:dbl)
        n106 = Subtract(x=w240, y=w238) -> (x-y=w237:dbl)
        n107 = Absolute Value(x=w237) -> (abs(x)=w235:dbl)
        n108 = Less?(x=2.0, y=w235) -> (x < y?=w259:bool)
        n109 = Not(x=w259) -> (.not. x?=w249:bool)
        n110 = case shown="True" w259 {
          tunnel: [0.0 w266] -> w264
          tunnel: w244 -> [_ w268]
          frame False {
          }
          frame True {
            n111 = Multiply(x=w268, y=0.4) -> (x*y=w266:dbl)
          }
        }
        n112 = Not Equal?(x=w247, y=0) -> (x != y?=w250:bool)
        n113 = Negate(x=w264) -> (-x=w263:dbl)
        n114 = And(x=w249, y=w250) -> (x .and. y?=w248:bool)
      }
      frame "Vision Turn" {
        w326 = 0.0 ("t")
        # "Record intial offset"
        # "If dist is < SD, and command hasnt just begun, finish"
        # "Flipped Left and right-Sarah"
        # "Fliipped"
        # "When we are to far off, we need to set the setpoint futher from the actualy gear target cetner, to make the robot over correct \nand curve in a circular way until the target is in the center. then, the normal taural program will begin"
        # "Is curving necessary?"
        # "TUNEEEEEE!!!!"
        # "*this will be true if score is less than 50"
        # "TODO: \nMake more robust. Make second cull and Group vi(scoring half a target) in Vision code\nwith priority on the original group vi for scoring a full target.\nAdd cases of taural program for only half a target.\nSince half the target is a little off from the center of the tru target, the p should be higher\nwhen dealing with only half a target(overshoot half target and recapture whole target)\n-switch p values by means of a bool passed trough a network table containing whether \n  or not rect is half or whole"
        # "Check Left or Right"
        # "If we loose the target\n, stop and wait"
        # "Start 7.775 ft (~7'9'') from the back of robot to the base of the gear peg"
        # "Left \nTop\nRight \nBottom"
        # "Gear Target Rectangle"
        n115 = global read "Drive Published Globals.vi" "Gear Rect"() -> (w324:T37)
        n116 = Unbundle(w324) -> ("Left"=w333:dbl, "Top"=w332:dbl, "Right"=w331:dbl, "Bottom"=w330:dbl)
        n117 = call "FindRectCenter.vi"("Bottom"=w330, "RIght"=w331, "Top"=w332, "Left"=w333) -> ("Y"=w297:dbl, "X"=w306:dbl)  [unwired: 6 in]
        n118 = Unbundle By Name(w320) -> ("Start Time (ms)"=w314:u32, "Iterations"=w285:i32)
        n119 = Divide(x="X resolution", y=2.0) -> (x/y=w305:dbl)
        n120 = Subtract(x=w306, y=w305) -> (x-y=w280:dbl)
        n121 = Less?(x=w285, y=5) -> (x < y?=w283:bool)
        n122 = Absolute Value(x=w280) -> (abs(x)=w287:dbl)
        "Vision P tuning threshold" <- w287
        n123 = Less?(x=w280, y=0.0) -> (x < y?=w302:bool)
        n124 = Subtract(x=w315, y=w314) -> (x-y=w313:u32)
        n125 = Less?(x=w285, y=50) -> (x < y?=w317:bool)
        n126 = Greater?(x=w287, y="Theshold for curve") -> (0:w282:bool)
        n127 = And(x=w283, y=w282) -> (x .and. y?=w281:bool)
        n128 = case shown="True" w281 {
          tunnel: w280 -> [_ w351]
          frame False {
          }
          frame True {
            n129 = global write "Drive Published Globals.vi" "Initial Offset"(w351) -> ()
          }
        }
        n130 = Not(x=w282) -> ()  [unwired: 1 out]
        n131 = Not(x=w317) -> (.not. x?=w286:bool)
        n132 = global read "Drive Published Globals.vi" "score"() -> (w288:dbl)
        n133 = case shown="True" TRUE {
          tunnel: [w356 w367] -> w304
          tunnel: w280 -> [w365 _]
          tunnel: w306 -> [w366 w367]
          tunnel: "X resolution" -> [w360 _]
          frame False {
            w362 = 0.0 ("y")
            # "Make sure imaginary center of target isn't\n negative or off screen? Is this necessary?\n Maybe its fine to have super far of targets"
            # "TUNEEEEEE!!!!"
            # "We want to\nmake the target seem\n futher off center"
            n134 = Multiply(x=w365, y="P curving factor") -> (x*y=w364:dbl)
            n135 = Add(x=w366, y=w364) -> (x+y=w357:dbl)
            n136 = Less?(x=w357, y=w362) -> (x < y?=w363:bool)
            n137 = Select(t=w362, s=w363, f=w357) -> (s? t:f=w359:dbl)
            n138 = Greater?(x=w359, y=w360) -> (0:w361:bool)
            n139 = Select(t=w360, s=w361, f=w359) -> (s? t:f=w356:dbl)
          }
          frame True {
            # "Normal Taural"
          }
        }
        n140 = Not Equal?(x=w288, y=0.0) -> (x != y?=w289:bool)
        n141 = Not Equal?(x=w288, y=-inf) -> (x != y?=w293:bool)
        n142 = Not Equal?(x=w288, y=inf) -> (x != y?=w292:bool)
        n143 = Compound Arithmetic op=AND(w289, w293, w292) -> (w290:bool)
        n144 = case shown="True" w290 {
          tunnel: w297 -> [_ w354]
          tunnel: [TRUE w353] -> w296
          frame False {
          }
          frame True {
            # "If target is below threshold, finish"
            n145 = Greater?(x=w354, y="Y stopping threshold") -> (0:w353:bool)
          }
        }
        n146 = call <vilib>:"WPI_AnalogChannelGetVoltage.vi"("AIDeviceRef"=w300) -> ("Voltage"=w269:dbl)  [unwired: 8 in, 2 out]
        "Voltage Graph" <- w269
        "Voltage now" <- w269
        n147 = Greater?(x=w269, y="Threshold voltage") -> (0:w298:bool)
        n148 = Compound Arithmetic op=AND(w298, w286, w296) -> (w325:bool)
        n149 = call-poly <vilib>:"NT Write Value.vi"("Numeric"=w269, "Name"="Voltage Now") -> ()  [unwired: 9 in, 1 out]
        n150 = case shown="False" w302 {
          tunnel: w304 -> [w376 w385]
          tunnel: w305 -> [w375 w384]
          tunnel: [w372 w382] -> w327
          tunnel: [w373 w381] -> w328
          tunnel: "Base Speed" -> [w371 w380]
          tunnel: "P Gear Tuner" -> [w374 w383]
          frame False {
            # "Left"
            # "Right"
            # "Error"
            # "Target is Right"
            n151 = Subtract(x=w376, y=w375) -> (x-y=w379:dbl)
            n152 = Divide(x=w379, y=w375) -> (x/y=w378:dbl)
            n153 = Multiply(x=w378, y=w374) -> (x*y=w377:dbl)
            n154 = Add(x=w371, y=w377) -> (x+y=w373:dbl)
            n155 = Subtract(x=w371, y=w377) -> (x-y=w372:dbl)
          }
          frame True {
            # "Left"
            # "Right"
            # "Error"
            # "Target is Left"
            n156 = Subtract(x=w384, y=w385) -> (x-y=w388:dbl)
            n157 = Divide(x=w388, y=w384) -> (x/y=w387:dbl)
            n158 = Multiply(x=w387, y=w383) -> (x*y=w386:dbl)
            n159 = Subtract(x=w380, y=w386) -> (x-y=w381:dbl)
            n160 = Add(x=w380, y=w386) -> (x+y=w382:dbl)
          }
        }
        n161 = Compound Arithmetic op=OR(FALSE ("Finish"), w325) -> (w319:bool)
        n162 = And(x=w319, y=w286) -> (x .and. y?=w310:bool)
        n163 = Greater?(x=w313, y=u32 6000) -> (0:w311:bool)
        n164 = Or(x=w310, y=w311) -> (x .or. y?=w301:bool)
        n165 = case shown="True" w301 {
          frame False {
            n166 = global write "Robot Global Data.vi" "Enable Vision"(TRUE ("Enable Vision")) -> ()
          }
          frame True {
            n167 = global write "Drive Published Globals.vi" "Initial Offset"(0.0 ("Initial Offset")) -> ()
            n168 = global write "Robot Global Data.vi" "Enable Vision"(FALSE ("Enable Vision")) -> ()
          }
        }
        n169 = global read "Drive Published Globals.vi" "score"() -> (w323:dbl)
        n170 = global read "Drive Published Globals.vi" "Initial Offset"() -> (w279:dbl)
        n171 = Less?(x=w323, y="Score Cutoff") -> (x < y?=w321:bool)
        n172 = Select(t=w326, s=w321, f=w328) -> (s? t:f=w277:dbl)
        n173 = Select(t=w326, s=w321, f=w327) -> (s? t:f=w275:dbl)
        n174 = Sign(1:w279) -> (0:w272:dbl)
        n175 = Absolute Value(x=w279) -> (abs(x)=w278:dbl)
        n176 = case shown="-1" w272 {
          tunnel: w277 -> [w338 w341 w350]
          tunnel: w278 -> [_ w344 w349]
          tunnel: [w338 w340 w350] -> w276
          tunnel: [w337 w339 w345] -> w274
          tunnel: w275 -> [w337 w339 w346]
          frame 0, Default {
            # "no offset"
          }
          frame 1 {
            # "Target is right"
            n177 = Multiply(x=w344, y="Fcurving left") -> (x*y=w342:dbl)
            n178 = Add(x=w342, y=w341) -> (x+y=w340:dbl)
          }
          frame -1 {
            # "Target Left"
            n179 = Multiply(x=w349, y="Fcurving right") -> (x*y=w347:dbl)
            n180 = Add(x=w347, y=w346) -> (x+y=w345:dbl)
          }
        }
        n181 = call-poly <vilib>:"NT Write Value.vi"("Numeric"=w272, "Name"="F Curving Mode") -> ()  [unwired: 9 in, 1 out]
      }
      frame "Turn until target" {
        n182 = global read "Drive Published Globals.vi" "score"() -> (w397:dbl)
        n183 = Not Equal?(x=w397, y=-inf) -> (x != y?=w399:bool)
        n184 = Not Equal?(x=w397, y=inf) -> (x != y?=w398:bool)
        n185 = Not Equal?(x=w397, y=0.0) -> (x != y?=w395:bool)
        n186 = Compound Arithmetic op=AND(w395, w399, w398) -> (w390:bool)
        n187 = Not(x=w390) -> (.not. x?=w389:bool)
        n188 = case shown="False" w389 {
          tunnel: [w402 0.3] -> w394
          tunnel: [w402 -0.3] -> w393
          frame False {
            w402 = 0.0
          }
          frame True {
          }
        }
      }
      frame "Brake" {
        w405 = WPI_SolenoidValue."On" ("Value")
        n189 = call-poly <vilib>:"WPI_SolenoidSet.vi"("Value"=w405, "SolenoidDevRef"=w406) -> ()  [unwired: 8 in, 2 out]
      }
      frame "DriveStraight" {
        # "feet"
        n190 = Unbundle(w436) -> ("Iterations"=w435:i32)  [unwired: 1 out]
        n191 = case shown="2" w435 {
          tunnel: w417 -> [w443 _ _ _]
          tunnel: w427 -> [w447 w449 w453 w459]
          tunnel: w426 -> [w446 w448 w452 w458]
          tunnel: [w445 w449 w453 w459] -> w420
          tunnel: [w444 w448 w452 w458] -> w424
          tunnel: w412 -> [_ _ w455 _]
          tunnel: w411 -> [_ _ w454 _]
          tunnel: [0.0 ("Left Setpoint") 0.0 ("Left Setpoint") w455 0.0 ("Left Setpoint")] -> w410
          tunnel: [0.0 ("Right Setpoint") 0.0 ("Right Setpoint") w454 0.0 ("Right Setpoint")] -> w409
          frame 0 {
            # "Reset Pigeon"
            n192 = call <vilib>:"CTRE_PigeonIMU_GetAll.vi"("PigeonIMUDevRef"=w443) -> ("Get All"=w442:T34)  [unwired: 8 in, 2 out]
            n193 = Unbundle By Name(w442) -> ("FusedHeading.Heading"=w441:dbl)
            n194 = call <vilib>:"WPI_EncoderReset.vi"("EncoderDevRef"=w446) -> ("EncoderDevRef"=w444:T21)  [unwired: 9 in, 1 out]
            n195 = call <vilib>:"WPI_EncoderReset.vi"("EncoderDevRef"=w447) -> ("EncoderDevRef"=w445:T21)  [unwired: 9 in, 1 out]
            n196 = global write "Drive Published Globals.vi" "pigeon"(w441) -> ()
          }
          frame 2 {
          }
          frame 3, Default {
          }
          frame 1 {
          }
        }
        n197 = call <vilib>:"WPI_EncoderGet.vi"("EncoderDevRef"=w424) -> ("Distance"=w423:dbl, "EncoderDevRef"=w419:T21)  [unwired: 5 in, 4 out]
        n198 = call <vilib>:"WPI_EncoderGet.vi"("EncoderDevRef"=w420) -> ("Distance"=w425:dbl)  [unwired: 5 in, 5 out]
        n199 = call <vilib>:"CTRE_PigeonIMU_GetAll.vi"("PigeonIMUDevRef"=w417) -> ("Get All"=w429:T34, "PigeonIMUDevRef"=w428:T30)  [unwired: 8 in, 1 out]
        n200 = Unbundle By Name(w429) -> ("FusedHeading.Heading"=w414:dbl)
        n201 = call "CheckEncoders.vi"("Target Distance"=w422, "Encoder Left"=w423, "Encoder Right"=w425) -> ("Distance Has Been Reached"=w421:bool)  [unwired: 8 in]
        n202 = global read "Drive Published Globals.vi" "pigeon"() -> (w413:dbl)
        n203 = Bundle("Heading"=w414, "pigeon"=w413) -> (→"Waveform Chart 2":cluster{"Heading":dbl, "\n\n\npigeon":dbl})  [unwired: 1 in]
        n204 = Subtract(x=w413, y=w414) -> (x-y=w416:dbl)
        n205 = Multiply(x=w416, y="PDriveStright") -> (x*y=w431:dbl)
        n206 = Add(x=w431, y=w410) -> (x+y=w432:dbl)
        n207 = Subtract(x=w409, y=w431) -> (x-y=w430:dbl)
        n208 = case shown="True" w421 {
          tunnel: w428 -> [_ _]
          tunnel: w420 -> [_ w438]
          tunnel: w419 -> [_ w437]
          frame False {
          }
          frame True {
            n209 = call <vilib>:"WPI_EncoderReset.vi"("EncoderDevRef"=w438) -> ()  [unwired: 9 in, 2 out]
            n210 = call <vilib>:"WPI_EncoderReset.vi"("EncoderDevRef"=w437) -> ()  [unwired: 9 in, 2 out]
          }
        }
      }
      frame "Drive for Distance" {
        n211 = Unbundle By Name(w483) -> ("Iterations"=w474:i32)  [unwired: 1 out]
        n212 = Multiply(x=w487, y=12.0) -> (x*y=w488:dbl)
        n213 = case shown="0" w474 {
          tunnel: w479 -> [w496 w498]
          tunnel: [w496 w497] -> w482
          frame 1, Default {
          }
          frame 0 {
            n214 = call <vilib>:"WPI_EncoderReset.vi"("EncoderDevRef"=w498) -> ("EncoderDevRef"=w497:T21)  [unwired: 9 in, 1 out]
          }
        }
        n215 = Multiply(x=3.5, y=3.141592653589793) -> (x*y=w490:dbl)
        n216 = case shown="0" w474 {
          tunnel: [w493 w495] -> w477
          tunnel: w478 -> [w493 w494]
          frame 1, Default {
          }
          frame 0 {
            n217 = call <vilib>:"WPI_EncoderReset.vi"("EncoderDevRef"=w494) -> ("EncoderDevRef"=w495:T21)  [unwired: 9 in, 1 out]
          }
        }
        n218 = Divide(x=w488, y=w490) -> (x/y=w486:dbl)
        n219 = Multiply(x="ticks per rotation", y=w486) -> (x*y=w473:dbl)
        n220 = call <vilib>:"WPI_EncoderGet.vi"("EncoderDevRef"=w482) -> ("Distance"=w465:dbl)  [unwired: 5 in, 5 out]
        n221 = call <vilib>:"WPI_EncoderGet.vi"("EncoderDevRef"=w477) -> ("Distance"=w466:dbl)  [unwired: 5 in, 5 out]
        n222 = Bundle("Distance"=w466, "Distance"=w465) -> (→"Waveform Chart":cluster{"Distance":dbl, "Distance":dbl})  [unwired: 1 in]
        n223 = Add(x=w465, y=w466) -> (x+y=w476:dbl)
        n224 = Divide(x=w476, y=2.0) -> (x/y=w463:dbl)
        n225 = Absolute Value(x=w463) -> (abs(x)=w460:dbl)
        n226 = call-poly <vilib>:"PID.vi"("output range"=cluster{"output high":dbl, "output low":dbl} {"output high"=1.0, "output low"=-1.0}, "PID gains"="PID gains", "process variable"=w460, "setpoint"=w473) -> ("output"=w464:dbl)  [unwired: 6 in, 1 out]
        n227 = Multiply(x=w464, y=w470) -> ()  [unwired: 1 out]
        n228 = Multiply(x=w464, y=w481) -> ()  [unwired: 1 out]
        n229 = Absolute Value(x=w464) -> (abs(x)=w468:dbl)
        n230 = Less?(x=w468, y="y") -> (x < y?=w461:bool)
        n231 = Multiply(x=w464, y=w470) -> (x*y=w462:dbl)
      }
      frame "Vision close distance" {
        n232 = call-poly <vilib>:"NT Read Value.vi"("Name"="Gear Distance") -> ("Numeric"=w504:dbl)  [unwired: 9 in, 1 out]
        n233 = Greater?(x=w504, y="Max dist") -> (0:w505:bool)
        n234 = case shown="True" w505 {
          tunnel: [TRUE FALSE] -> w502
          tunnel: [0.0 0.2] -> w500
          frame False {
          }
          frame True {
          }
        }
      }
    }
    n235 = local read "Threshold voltage"() -> (w91:dbl)
    n236 = call-poly <vilib>:"NT Read Value.vi"("Default Value"=w91, "Name"="Threshold voltage") -> ("Numeric"=w90:dbl)  [unwired: 8 in, 1 out]
    n237 = local write "Threshold voltage"(w90) -> ()
    n238 = local read "Fcurving left"() -> (w97:dbl)
    n239 = call-poly <vilib>:"NT Read Value.vi"("Default Value"=w97, "Name"="F Curving Left") -> ("Numeric"=w96:dbl)  [unwired: 8 in, 1 out]
    n240 = local write "Fcurving left"(w96) -> ()
    n241 = local read "Fcurving right"() -> (w94:dbl)
    n242 = call-poly <vilib>:"NT Read Value.vi"("Default Value"=w94, "Name"="F Curving Right") -> ("Numeric"=w95:dbl)  [unwired: 8 in, 1 out]
    n243 = local write "Fcurving right"(w95) -> ()
    n244 = call <vilib>:"WPI_RobotDriveMotors.vi"("RightSpeed"=w124, "LeftSpeed"=w125, "RobotDriveDevRef"=w106) -> ()  [unwired: 1 in, 8 out]
    n245 = Bundle("t"=w125, "t"=w124) -> (→"Setpoints":cluster{"t":dbl, "t":dbl})  [unwired: 1 in]
    n246 = call "Drive Check for New Command.vi"("input cluster"=w110, "Wait time (ms)"=w115, "Finished?"=w101) -> ("Completion"=w117:T27, "Subsystem Name"=w112:string, "SetPoint"=w113:T9, "Initial Trace String"=w114:string, "output cluster"=w116:T38)  [unwired: 4 in]
    n247 = case shown="\"Successful\", \"Aborted\"" w117 {
      selector: w117 -> [_ w142]
      tunnel: w114 -> [_ w137]
      tunnel: w113 -> [_ w138]
      tunnel: w112 -> [_ w135]
      tunnel: w101 -> [_ w132]
      frame "Incomplete", Default {
        # "Continuing current command"
      }
      frame "Successful", "Aborted" {
        # "Report and setup for next command"
        n248 = Unbundle By Name(w138) -> ("Left Setpoint"=w140:dbl, "Right Setpoint"=w141:dbl, "Duration"=w136:dbl)
        n249 = case shown="True" w132 {
          tunnel: ["Bad" "Finish"] -> w131
          frame False {
          }
          frame True {
          }
        }
        n250 = Format Into String(format string="L %.1f, R %.1f, D %f", initial string=w137, w140, w141, w136) -> (resulting string=w129:string)  [unwired: 1 in, 1 out]
        "Current\nCmd" <- w129
        n251 = call <vilib>:"Trace Results.vi"("Status of previous command"=w142, "Description"=w129, "Subsystem"=w135) -> ()  [unwired: 9 in]
        n252 = Concatenate Strings(w131, w129) -> (w130:string)
        n253 = call <vilib>:"WPI_DriverStationGetModeAndStatus.vi"() -> ("Robot Mode"=w133:T39)  [unwired: 10 in, 1 out]
        n254 = call-poly <vilib>:"NT Write Value.vi"("String"=w129, "Name"="Current Drive") -> ()  [unwired: 9 in, 1 out]
        n255 = case shown="\"Autonomous Enabled\"" w133 {
          tunnel: w130 -> [_ w145]
          frame "Autonomous Disabled", Default {
          }
          frame "Autonomous Enabled" {
            n256 = call <vilib>:"NetComm_SendMessage.vi"("Message"=w145) -> ()  [unwired: 11 in]
          }
        }
      }
    }
  }
